vi "GageAvgSpec_test.vi"() -> ()   [LabVIEW 2016]
panel:
  out "Sample Bits 2":i32
  out "Board Count 2":i32
  out "Channel Count 2":i32
  out "Trigger Count 2":i32
  out "System Name 2":string
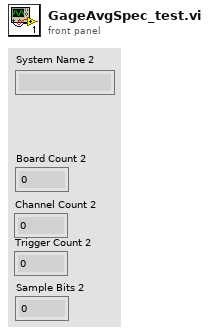
[diagram p1: front panel]
types:
  T1 = cluster{"Handle":u32, "Sample size":u32, "Resolution":i32, "Offset":i32, "Channels":u32, "Boards":u32}
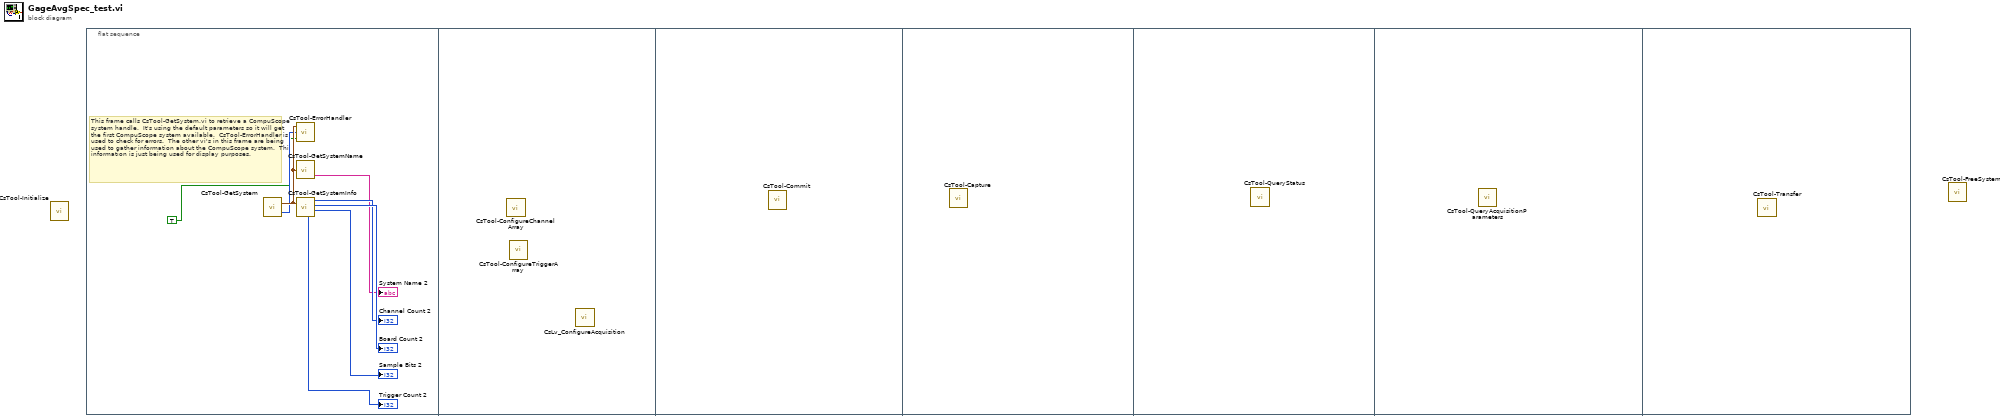
[diagram p0: block diagram]
diagram:
  n1 = call "CsTool-Initialize.vi"() -> ()  [unwired: 2 out]
  n2 = flat-sequence {
    frame #0 {
      # "This frame calls CsTool-GetSystem.vi to retrieve a CompuScope system handle.  It's using the default parameters so it will get the first CompuScope system available.  CsTool-ErrorHandler is used to check for errors.  The other vi's in this frame are being used to gather information about the CompuScope system.  This information is just being used for display purposes."
      n3 = call "CsTool-GetSystem.vi"() -> ("Error Code"=w5:i32, "Handle Cluster"=w6:T1)  [unwired: 4 in]
      n4 = call "CsTool-ErrorHandler.vi"("StopOnError (true)"=TRUE, "Error Code"=w5, "Handle Cluster"=w6) -> ()  [unwired: 1 out]
      n5 = call "CsTool-GetSystemName.vi"("Handle Cluster"=w6) -> ("System Name"=→"System Name 2":string)  [unwired: 1 out]
      n6 = call "CsTool-GetSystemInfo.vi"("Handle Cluster"=w6) -> ("Number Of Triggers"=→"Trigger Count 2":u32, "Number Of Channels"=→"Channel Count 2":u32, "Number Of Boards"=→"Board Count 2":u32, "Sample Bits"=→"Sample Bits 2":u32)  [unwired: 3 out]
    }
    frame #1 {
      n7 = call "CsTool-ConfigureChannelArray.vi"() -> ()  [unwired: 2 in, 1 out]
      n8 = call "CsTool-ConfigureTriggerArray.vi"() -> ()  [unwired: 2 in, 1 out]
      n9 = call "CsLv_ConfigureAcquisition.vi"() -> ()  [unwired: 11 in, 1 out]
    }
    frame #2 {
      n10 = call "CsTool-Commit.vi"() -> ()  [unwired: 3 in, 2 out]
    }
    frame #3 {
      n11 = call "CsTool-Capture.vi"() -> ()  [unwired: 1 in, 1 out]
    }
    frame #4 {
      n12 = call "CsTool-QueryStatus.vi"() -> ()  [unwired: 1 in, 1 out]
    }
    frame #5 {
      n13 = call "CsTool-QueryAcquisitionParameters.vi"() -> ()  [unwired: 1 in, 11 out]
    }
    frame #6 {
      n14 = call "CsTool-Transfer.vi"() -> ()  [unwired: 6 in, 4 out]
    }
  }
  n15 = call "CsTool-FreeSystem.vi"() -> ()  [unwired: 1 in, 1 out]
